vi "svc_Convert Spectrum Cluster to X and Y Arrays.vi"(7 "spectrum":cluster{"x0":dbl, "dx":dbl, "Y":dbl[]}={"x0"=0.0, "dx"=1.0, "Y"=[]}) -> (6 "X":dbl[](array[numeric]), 10 "Y":dbl[](array[numeric]))   [LabVIEW 2017]
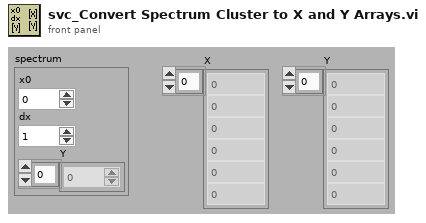
[diagram p1: front panel]
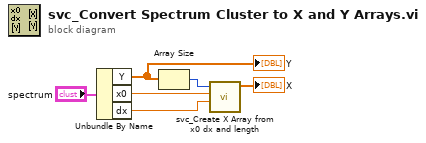
[diagram p0: block diagram]
diagram:
  n1 = Unbundle By Name("spectrum") -> ("Y"=w5:dbl[], "x0"=w4:dbl, "dx"=w1:dbl)
  "Y" <- w5
  n2 = Array Size(array=w5) -> (size(s)=w3:i32)
  n3 = call <vilib>:"svc_Create X Array from x0 dx and length.vi"("dx"=w1, "x0"=w4, "length"=w3) -> ("X"=→"X":dbl[])  [unwired: 8 in]
